vi "Is Valid Item.vi"(8 "error in (no error)":errorcluster, 10 "Item ID":string, 11 "Item in":refnum<class "Item.lvclass">) -> (0 "error out":errorcluster, 1 "Is Valid?":bool, 2 "Is Item?":bool, 3 "Item out":refnum<class "Item.lvclass">)   [LabVIEW 2020, in "VI Properties Editor.lvlib" / "Item.lvclass"]
doc: "Checks if <B>Item in</B> is identified by <B>Item ID</B> and checks if it is a valid item, meaning one that is able to be edited in the application."
uses:
  Item.lvclass
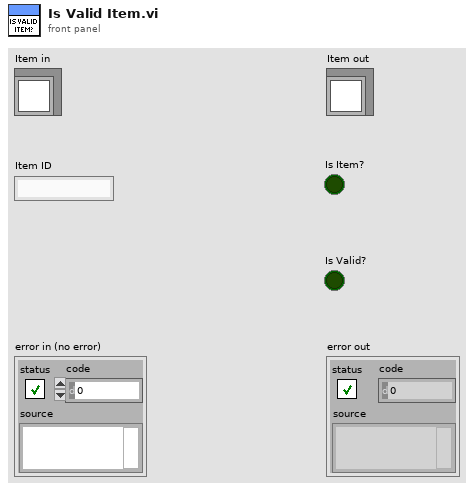
[diagram p1: front panel]
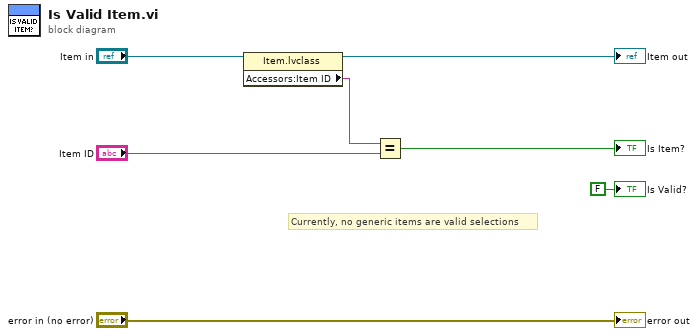
[diagram p0: block diagram]
diagram:
  # "Currently, no generic items are valid selections"
  n1 = property class="Item.lvclass"(reference="Item in") -> (reference out=→"Item out":refnum<class "Item.lvclass">, "Accessors:Item ID"=w2:string)  [unwired: 1 in, 1 out]
  n2 = Equal?(x=w2, y="Item ID") -> (x = y?=→"Is Item?":bool)
  "error out" <- "error in (no error)"
  "Is Valid?" <- FALSE ("Is Valid?")
